vi "Unpack Subscription Request.vi"(11 "SubscriptionRequest in":refnum<class "SubscriptionRequest.lvclass">) -> (0 "Transport":refnum<class "ITransport.lvclass">, 1 "Unique Subscriber ID":string, 2 "Type":variant, 3 "Topic Name":string, 4 "SubscriptionPolicy":refnum<class "SubscriptionPolicy.lvclass">)   [LabVIEW 2015, in "IMediator.lvlib" / "SubscriptionRequest.lvclass"]
doc: "<License>\nCopyright © 2017 Composed Systems, LLC | All rights reserved\nwww.composed.io\n\nAuthor: Ethan Stern <ethan.stern@composed.io>\n\nThis software is provided \"AS IS\" WITHOUT WARRANTIES, either express or implied, AND IS FOR EDUCATIONAL PURPOSES ONLY.\n</License>"
uses:
  SubscriptionRequest.lvclass
  ITransport/ITransport.lvclass
  SubscriptionPolicy/SubscriptionPolicy.lvclass
  SubscriptionRequest.lvclass/SubscriptionRequest.ctl
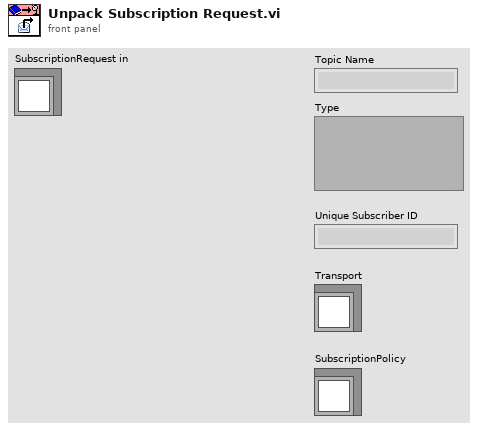
[diagram p1: front panel]
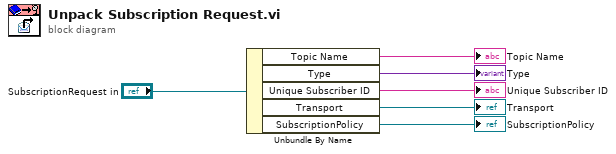
[diagram p0: block diagram]
diagram:
  n1 = Unbundle By Name("SubscriptionRequest in") -> ("Topic Name"=→"Topic Name":string, "Type"=→"Type":variant, "Unique Subscriber ID"=→"Unique Subscriber ID":string, "Transport"=→"Transport":refnum<class "ITransport.lvclass">, "SubscriptionPolicy"=→"SubscriptionPolicy":refnum<class "SubscriptionPolicy.lvclass">)
